vi "CreateProcces.vi"(0 "reference in":refnum<class "Proccess.lvclass">, 5 "error in (no error)":errorcluster, 12 "Tags":T1, 13 "Logger":refnum<class "Logger.lvclass">) -> (14 "reference out":refnum<class "Proccess.lvclass">, 19 "error out":errorcluster)   [LabVIEW 2019, in "Proccess.lvclass"]
doc: "Constructor."
uses:
  Proccess.lvclass
  Logger_class/Logger.lvclass
  TAGs.ctl
  Proccess.lvclass/Proccess.ctl
  Logger_class/ObjData.ctl
  Logger_class/ObjType.ctl
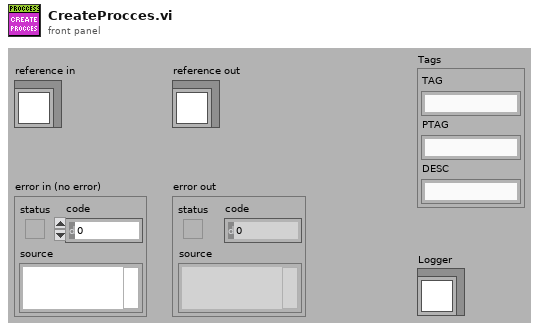
[diagram p1: front panel]
types:
  T1 = typedef "Proccess.lvclass/TAGs.ctl" = cluster{"TAG":string, "PTAG":string, "DESC":string}
  T2 = typedef "Logger.lvclass/ObjType.ctl" = enum16{"Procces", "Device", "Signal", "DI", "DO", "DA", "AI", "AO", "AA"}
  T3 = typedef "Logger.lvclass/ObjData.ctl" = cluster{"object_tag":string, "parent_tag":string, "object_type":T2, "description":string}
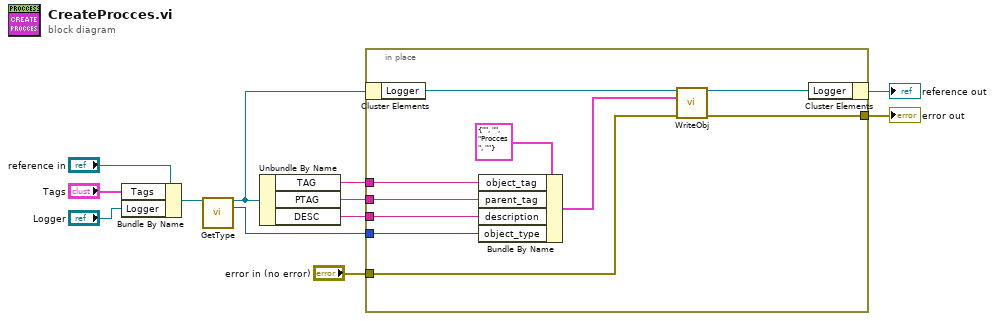
[diagram p0: block diagram]
diagram:
  n1 = Bundle By Name(cluster="reference in", "Tags"="Tags", "Logger"="Logger") -> (w10:refnum<class "Proccess.lvclass">)
  n2 = call-dynamic "GetType.vi"("reference in"=w10) -> ("reference out"=w6:refnum<class "Proccess.lvclass">, "obj_type"=w7:T2)  [unwired: 13 in]
  n3 = Unbundle By Name(w6) -> ("TAG"=w9:string, "PTAG"=w8:string, "DESC"=w5:string)
  n4 = in-place {
    in-place-border: w9 -> [w18]
    in-place-border: w8 -> [w17]
    in-place-border: w7 -> [w16]
    in-place-border: w5 -> [w15]
    in-place-border: "error in (no error)" -> [w14]
    in-place-border: [w13] -> w4
    n5 = in-place-cluster #1(w6) -> ("Logger"=w21:refnum<class "Logger.lvclass">)
    n6 = Bundle By Name(cluster=T3 {"object_tag"="", "parent_tag"="", "object_type"=enum."Procces", "description"=""} ("device"), "object_tag"=w18, "parent_tag"=w17, "description"=w15, "object_type"=w16) -> (w19:T3)
    n7 = call "WriteObj.vi"("reference in"=w21, "device"=w19, "error in (no error)"=w14) -> ("reference out"=w20:refnum<class "Logger.lvclass">, "error out"=w13:errorcluster)  [unwired: 11 in]
    n8 = in-place-cluster #1("Logger"=w20) -> (→"reference out":refnum<class "Proccess.lvclass">)
  }
  "error out" <- w4
